vi "例7-4(1).vi"() -> ()   [LabVIEW 2019]
uses:
  <vilib>/Analysis/NI_AALBase.lvlib
panel:
  in  "停止按钮":bool
  in  "远程计算机地址":string="LocalHost"
  in  "远地端口":dbl=65511.0
  in  "本地端口":dbl=65510.0
  out "波形图（服务器）":dbl[](graph)
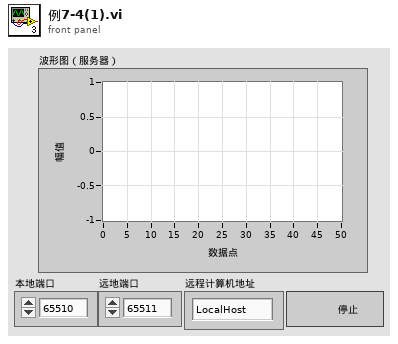
[diagram p1: front panel]
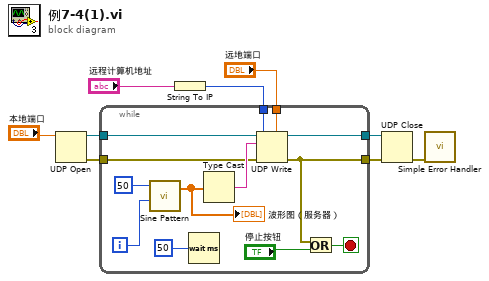
[diagram p0: block diagram]
diagram:
  n1 = UDP Open(11:"本地端口") -> (port=w7:refnum<k16>, 0:w2:errorcluster)  [unwired: 4 in, 1 out]
  n2 = String To IP(1:"远程计算机地址") -> (0:w4:u32)
  n3 = while {
    tunnel: w7 -> [w22]
    tunnel: "远地端口" -> [w17]
    tunnel: w4 -> [w16]
    tunnel: [w15] -> w3
    tunnel: w2 -> [w13]
    tunnel: [w12] -> w1
    i -> [w20]
    stop <- w14 stop-if-true
    n4 = call <vilib>:"Sine Pattern.vi"("phase(degrees)"=w20, "samples"=50) -> ("Sinusoidal Pattern"=w18:dbl[])  [unwired: 2 in, 1 out]
    "波形图（服务器）" <- w18
    n5 = Wait (ms)(milliseconds to wait=50) -> ()  [unwired: 1 out]
    n6 = Type Cast(x=w18) -> (*(type *) &x=w19:string)  [unwired: 1 in]
    n7 = UDP Write(address=w16, port or service name=w17, connection ID=w22, data in=w19, 8:w13) -> (error out=w12:errorcluster, 3:w15:refnum<k16>)  [unwired: 1 in]
    n8 = Or(x=w12, y="停止按钮") -> (x .or. y?=w14:bool)
  }
  n9 = UDP Close(connection ID=w3, 8:w1) -> (error out=w9:errorcluster)  [unwired: 1 out]
  n10 = call <vilib>:"Simple Error Handler.vi"("error in (no error)"=w9) -> ()  [unwired: 4 in, 5 out]
